vi "ws_testing search for sequence.vi"(4 "Test Station? (f)":bool, 6 "User":T3, 7 "httpRequestID":u32, 8 "error in (no error)":errorcluster, 9 "TestSeqId (\"\")":string, 10 "Action (\"Search\")":string="Search", 11 "Connection Refnum":T1) -> (0 "error out":errorcluster, 1 "Template Keys":T2, 2 "Template":string, 3 "Connection Refnum":T1)   [LabVIEW 2011]
uses:
  server/database/Users/User Record.ctl
  <vilib>/addons/internet/utils/keyedarr.llb/Keyed Array.ctl
  SI.LIB/ODBC/SQL Controls/Connection Refnum.ctl
  <vilib>/addons/internet/utils/strutil.llb/Case Matching.ctl
  <vilib>/wsapi/NI_WebServices.lvlib
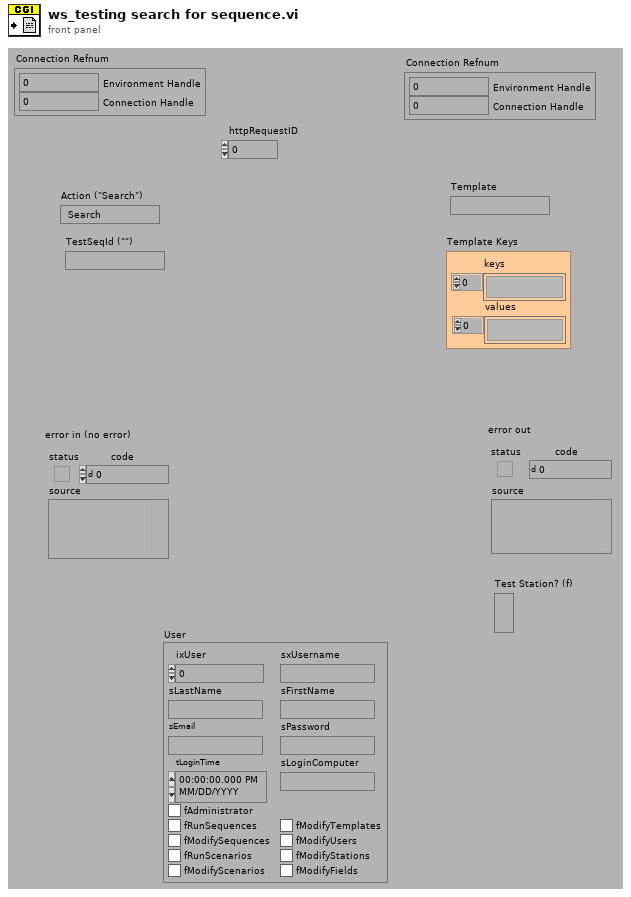
[diagram p1: front panel]
types:
  T1 = typedef "Connection Refnum.ctl" = cluster{"Environment Handle":i32, "Connection Handle":i32}
  T2 = typedef "Keyed Array.ctl" = cluster{"keys":string[], "values":string[]}
  T3 = typedef "User Record.ctl" = cluster{"ixUser":i32, "sxUsername":string, "sLastName":string, "sFirstName":string, "sEmail":string, "sPassword":string, "tLoginTime":timestamp, "sLoginComputer":string, "fAdministrator":bool, "fRunSequences":bool, "fModifySequences":bool, "fRunScenarios":bool, "fModifyScenarios":bool, "fModifyTemplates":bool, "fModifyUsers":bool, "fModifyStations":bool, "fModifyFields":bool}
  T4 = typedef "Sequence Record.ctl" = cluster{"ixSequence":i32, "sxSequenceId":string, "sDescription":string, "sCreator":string, "tCreationDate":timestamp, "sModifier":string, "tModifiedDate":timestamp, "fApproved":bool, "fSpartanSetsSN":bool, "fOverwriteData":bool, "fStopOnFail":bool, "fDisableQuickMode":bool, "fPartialExecution":bool, "fAutoNextItem":bool, "fDoNotPrintOnFail":bool}
  T5 = typedef "Case Matching.ctl" = enum16{"a != A", "a == A", "system"}
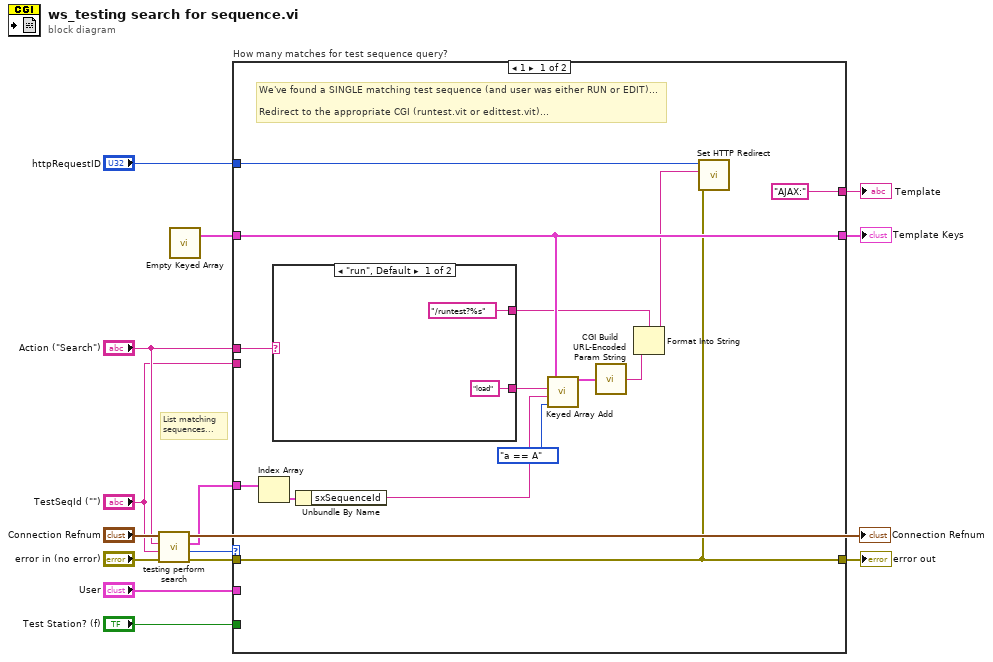
[diagram p0: block diagram]
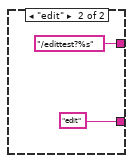
[diagram p2: hidden frame]
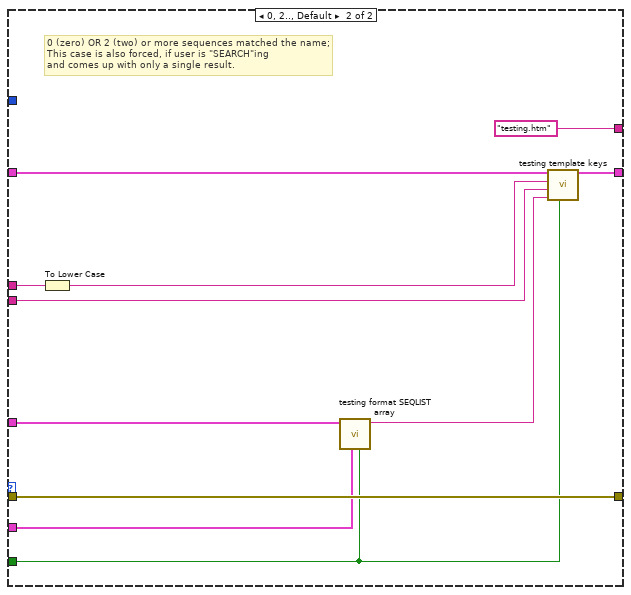
[diagram p3: hidden frame]
diagram:
  # "List matching\nsequences..."
  n1 = call "testing perform search.vi"("error in (no error)"="error in (no error)", "TestSeqId (\"\")"="TestSeqId (\"\")", "Action (\"Search\")"="Action (\"Search\")", "Connection Refnum"="Connection Refnum") -> ("error out"=w3:errorcluster, "Matching Results"=w4:i32, "Results"=w5:T4[], "Connection Refnum"=→"Connection Refnum":T1)  [unwired: 1 in, 3 out]
  n2 = call "Empty Keyed Array.vi"() -> ("empty keyed array"=w12:T2)  [unwired: 3 out]
  n3 = case "How many matches for test sequence query?" shown="1" w4 {
    tunnel: "TestSeqId (\"\")" -> [_ w37]
    tunnel: w5 -> [w27 w42]
    tunnel: "User" -> [_ w34]
    tunnel: [w28 w40] -> w15
    tunnel: w12 -> [w28 w36]
    tunnel: w3 -> [w17 w44]
    tunnel: [w17 w44] -> w14
    tunnel: ["AJAX:" "testing.htm" ("key")] -> w13
    tunnel: "Action (\"Search\")" -> [w20 w43]
    tunnel: "httpRequestID" -> [w18 _]
    tunnel: "Test Station? (f)" -> [_ w35]
    frame 1 {
      # "We've found a SINGLE matching test sequence (and user was either RUN or EDIT)...\n\nRedirect to the appropriate CGI (runtest.vit or edittest.vit)..."
      n4 = Index Array(array=w27) -> (element=w29:T4)  [unwired: 1 in]
      n5 = case shown="\"run\", Default" w20 {
        tunnel: ["load" ("key") "edit" ("key")] -> w21
        tunnel: ["/runtest?%s" ("New URL (/cgi-bin/testing.vit)") "/edittest?%s" ("New URL (/cgi-bin/testing.vit)")] -> w19
        frame "run", Default {
        }
        frame "edit" {
        }
      }
      n6 = Unbundle By Name(w29) -> ("sxSequenceId"=w22:string)
      n7 = call <vilib>:"Keyed Array Add.vi"("case matching (sensitive)"=Case_Matching."a == A", "value"=w22, "key"=w21, "array in"=w28) -> ("array out"=w24:T2)  [unwired: 1 in, 2 out]
      n8 = call <vilib>:"CGI Build URL-Encoded Param String.vi"("params"=w24) -> ("url-encoded param string"=w23:string)
      n9 = Format Into String(format string=w19, w23) -> (resulting string=w16:string)  [unwired: 2 in, 1 out]
      n10 = call <vilib>:"Set HTTP Redirect.vi"("error in (no error)"=w17, "redirect URL"=w16, "httpRequestID"=w18) -> ()  [unwired: 7 in, 2 out]
    }
    frame 0, 2.., Default {
      # "0 (zero) OR 2 (two) or more sequences matched the name;\nThis case is also forced, if user is \"SEARCH\"ing\nand comes up with only a single result."
      n11 = To Lower Case(string=w43) -> (all lower case string=w39:string)
      n12 = call "testing format SEQLIST array.vi"("Test Station? (f)"=w35, "User Information"=w34, "Results"=w42) -> ("SEQLIST array"=w38:string)  [unwired: 8 out]
      n13 = call "testing template keys.vi"("Test Station? (f)"=w35, "$$SEQLIST$$ (\"\")"=w38, "$$SEQID$$ (\"\")"=w37, "$$MODE$$ (\"\")"=w39, "Keys In"=w36) -> ("Keys Out"=w40:T2)  [unwired: 1 in, 5 out]
    }
  }
  "error out" <- w14
  "Template Keys" <- w15
  "Template" <- w13
